vi "DecodeCluster.vi"(8 "error in (no error)":errorcluster, 10 "TimeZone":i32, 11 "value":T1) -> (0 "error out":errorcluster, 2 "time stamp":timestamp, 3 "USD":dbl format="%#_15g")   [LabVIEW 2017, in "WebRead.lvlib"]
uses:
  WebRead.lvlib
  ctl/JSONForm.ctl
  <vilib>/Utility/miscctls.llb/LVDateTimeRec.ctl
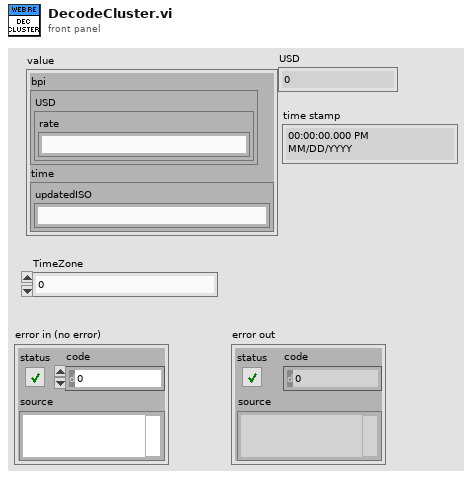
[diagram p1: front panel]
types:
  T1 = typedef "WebRead.lvlib/JSONForm.ctl" = cluster{"bpi":cluster{"USD":cluster{"rate":string}}, "time":cluster{"updatedISO":string}}
  T2 = typedef "LVDateTimeRec.ctl" = cluster{"fractional second":dbl, "second":i32, "minute":i32, "hour":i32, "day of month":i32, "month":i32, "year":i32, "day of week":i32, "day of year":i32, "DST":i32}
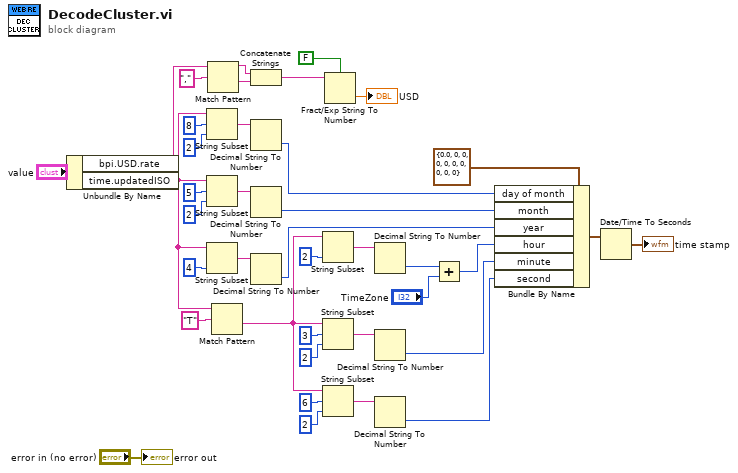
[diagram p0: block diagram]
diagram:
  n1 = Unbundle By Name("value") -> ("bpi.USD.rate"=w10:string, "time.updatedISO"=w24:string)
  n2 = String Subset(string=w24, offset (0)=8 ("length (rest)"), length (rest)=2 ("length (rest)")) -> (substring=w28:string)
  n3 = String Subset(string=w24, offset (0)=5 ("length (rest)"), length (rest)=2 ("length (rest)")) -> (substring=w30:string)
  n4 = String Subset(string=w24, length (rest)=4 ("length (rest)")) -> (substring=w35:string)  [unwired: 1 in]
  n5 = Match Pattern(string=w10, regular expression="," ("substring (\"\")")) -> (before substring=w8:string, after substring=w7:string)  [unwired: 1 in, 2 out]
  n6 = Match Pattern(string=w24, regular expression="T") -> (after substring=w13:string)  [unwired: 1 in, 3 out]
  n7 = Concatenate Strings(w8, w7) -> (w6:string)
  n8 = Decimal String To Number(string=w28) -> (number=w25:i32)  [unwired: 2 in, 1 out]
  n9 = Decimal String To Number(string=w30) -> (number=w29:i32)  [unwired: 2 in, 1 out]
  n10 = Decimal String To Number(string=w35) -> (number=w33:i32)  [unwired: 2 in, 1 out]
  n11 = String Subset(string=w13, length (rest)=2 ("length (rest)")) -> (substring=w21:string)  [unwired: 1 in]
  n12 = String Subset(string=w13, offset (0)=3 ("length (rest)"), length (rest)=2 ("length (rest)")) -> (substring=w20:string)
  n13 = String Subset(string=w13, offset (0)=6 ("length (rest)"), length (rest)=2 ("length (rest)")) -> (substring=w14:string)
  n14 = Fract/Exp String To Number(use system decimal point (T)=FALSE, string=w6) -> (number=→"USD":dbl)  [unwired: 2 in, 1 out]
  n15 = Decimal String To Number(string=w21) -> (number=w3:i32)  [unwired: 2 in, 1 out]
  n16 = Decimal String To Number(string=w20) -> (number=w17:i32)  [unwired: 2 in, 1 out]
  n17 = Decimal String To Number(string=w14) -> (number=w12:i32)  [unwired: 2 in, 1 out]
  n18 = Add(x=w3, y="TimeZone") -> (x+y=w2:i32)
  n19 = Bundle By Name(cluster=T2 {"fractional second"=0.0, "second"=0, "minute"=0, "hour"=0, "day of month"=0, "month"=0, "year"=0, "day of week"=0, "day of year"=0, "DST"=0} ("date time rec"), "day of month"=w25, "month"=w29, "year"=w33, "hour"=w2, "minute"=w17, "second"=w12) -> (w37:T2)
  n20 = Date/Time To Seconds(2:w37) -> (0:→"time stamp":timestamp)  [unwired: 1 in]
  "error out" <- "error in (no error)"
